vi "RSD.vi"(2 "S":bool, 3 "C":bool, 4 "D":bool, 5 "R":bool) -> (0 "Q2":bool, 1 "Q1":bool)   [LabVIEW 2013]
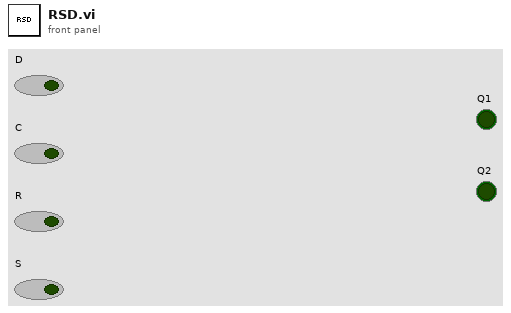
[diagram p1: front panel]
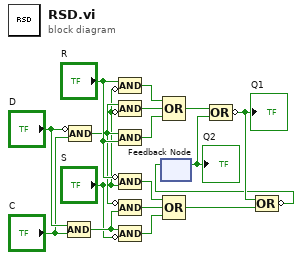
[diagram p0: block diagram]
diagram:
  n1 = Compound Arithmetic op=AND("D", "C") -> (w14:bool)
  n2 = Compound Arithmetic op=AND(invert "D", "C") -> (w13:bool)
  n3 = Compound Arithmetic op=AND("R", invert "S") -> (w11:bool)
  n4 = Compound Arithmetic op=AND(w13, invert "S") -> (w10:bool)
  n5 = Compound Arithmetic op=AND(w13, "R") -> (w9:bool)
  n6 = Compound Arithmetic op=AND(invert "R", "S") -> (w8:bool)
  n7 = Compound Arithmetic op=AND(invert w13, w14) -> (w7:bool)
  n8 = Compound Arithmetic op=AND(w14, invert "S") -> (w6:bool)
  n9 = feedback #1() -> (w1:bool)  [unwired: 1 in]
  "Q2" <- w1
  n10 = Compound Arithmetic op=OR(w11, w10, w9) -> (w5:bool)
  n11 = Compound Arithmetic op=OR(w8, w7, w6) -> (w4:bool)
  n12 = Compound Arithmetic op=OR(w5, w1) -> (invert w3:bool)
  "Q1" <- w3
  n13 = Compound Arithmetic op=OR(w3, w4) -> (invert w2:bool)
  n14 = feedback-in #1(w2) -> ()
